vi "Calculo_do_Azimute_da_Cupula_2.vi"(4 "AplicarAjuste":bool=TRUE, 5 "AH":dbl, 6 "DEC":dbl, 7 "OffsetTCSPD":dbl) -> (2 "PosCup":u16, 3 "Saída Cód Barras":string)   [LabVIEW 2018]
uses:
  Global_Telescopio.vi
panel:
  out "AngCupAjustado":dbl
  out "AngCup":dbl
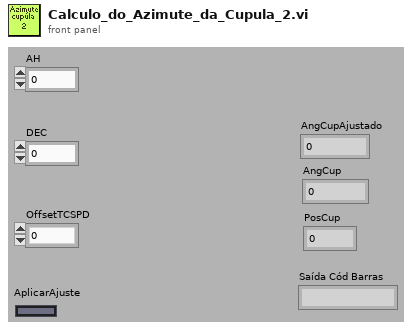
[diagram p1: front panel]
types:
  T1 = cluster{"QtdEtiq":u16, "EtiqMin":u16, "EtiqMax":u16, "Offset":dbl, "SegurancaAjuste":dbl, "LargTrapeira":dbl, "ProjecaoTubo":dbl, "RaioCupula":dbl, "DistEntreEixos":dbl, "AltBase":dbl, "LATrad":dbl}
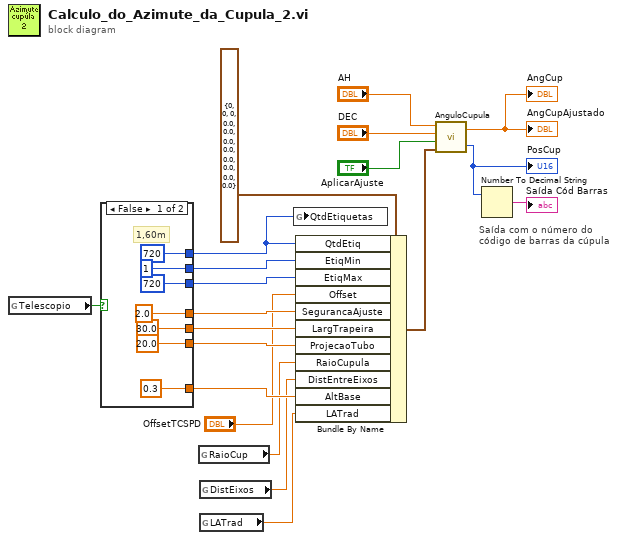
[diagram p0: block diagram]
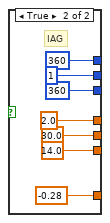
[diagram p2: hidden frame]
diagram:
  # "Saída com o número do\ncódigo de barras da cúpula"
  n1 = global read "Global_Telescopio.vi" "Telescopio"() -> (w2:bool)
  n2 = case shown="False" w2 {
    tunnel: [0.3 ("AltBase") -0.28 ("AltBase")] -> w14
    tunnel: [20.0 ("ProjecaoTubo") 14.0 ("ProjecaoTubo")] -> w11
    tunnel: [30.0 ("LargTrapeira") 30.0 ("LargTrapeira")] -> w10
    tunnel: [2.0 ("SegurancaAjuste") 2.0 ("SegurancaAjuste")] -> w9
    tunnel: [u16 720 ("EtiqMax") u16 360 ("EtiqMax")] -> w8
    tunnel: [u16 1 ("EtiqMin") u16 1 ("EtiqMin")] -> w7
    tunnel: [u16 720 ("QtdEtiq") u16 360 ("QtdEtiq")] -> w1
    frame False {
      # "1,60m"
    }
    frame True {
      # "IAG"
    }
  }
  n3 = global read "Global_Telescopio.vi" "RaioCup"() -> (w12:dbl)
  n4 = global read "Global_Telescopio.vi" "DistEixos"() -> (w13:dbl)
  n5 = global read "Global_Telescopio.vi" "LATrad"() -> (w15:dbl)
  n6 = global write "Global_Telescopio.vi" "QtdEtiquetas"(w1) -> ()
  n7 = Bundle By Name(cluster=T1 {"QtdEtiq"=0, "EtiqMin"=0, "EtiqMax"=0, "Offset"=0.0, "SegurancaAjuste"=0.0, "LargTrapeira"=0.0, "ProjecaoTubo"=0.0, "RaioCupula"=0.0, "DistEntreEixos"=0.0, "AltBase"=0.0, "LATrad"=0.0} ("ConstantesCupTel"), "QtdEtiq"=w1, "EtiqMin"=w7, "EtiqMax"=w8, "Offset"="OffsetTCSPD", "SegurancaAjuste"=w9, "LargTrapeira"=w10, "ProjecaoTubo"=w11, "RaioCupula"=w12, "DistEntreEixos"=w13, "AltBase"=w14, "LATrad"=w15) -> (w16:T1)
  n8 = call "AnguloCupula.vi"("ConstantesCupTel"=w16, "AplicarAjuste"="AplicarAjuste", "DEC"="DEC", "AH"="AH") -> ("PosCup"=w4:u16, "AngCup"=→"AngCup" →"AngCupAjustado":dbl)
  "PosCup" <- w4
  n9 = Number To Decimal String(number=w4) -> (decimal integer string=→"Saída Cód Barras":string)  [unwired: 1 in]
